vi "Read_Traverse_Space_Size.vi"(1 "Space_Name":string, 2 "Traverse Name":string) -> (0 "Limits out":T1=[{"Max"=15.0, "Min"=-15.0}, {"Max"=250.0, "Min"=0.0}, {"Max"=15.0, "Min"=-15.0}] {"Min" format="%#.1f"; "Max" format="%#.1f"})   [LabVIEW 2022 SP3]
uses:
  Route mapping/Box_size.ctl
  Globals/Constants_global.vi
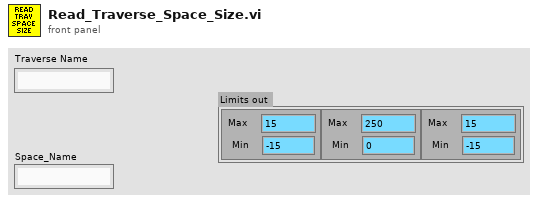
[diagram p1: front panel]
types:
  T1 = typedef "Box_size.ctl" = cluster{"Max":sgl, "Min":sgl}[]
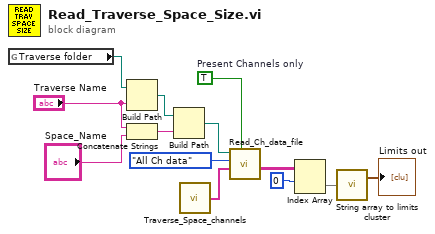
[diagram p0: block diagram]
diagram:
  w8 = TRUE  # Present Channels only
  n1 = global read "Constants_global.vi" "Traverse folder"() -> (w6:path)
  n2 = Build Path(base path=w6, name or relative path="Traverse Name") -> (appended path=w5:path)
  n3 = Concatenate Strings("Traverse Name", "Space_Name") -> (w9:string)
  n4 = Build Path(base path=w5, name or relative path=w9) -> (appended path=w10:path)
  n5 = call "Traverse_Space_channels.vi"() -> ("Channel Names"=w3:string[])
  n6 = call "Read_Ch_data_file.vi"("Present Channels only"=w8, "Present Channels"=w3, "Output"=enum16{"All Ch data", "The last few rows"}."All Ch data", "Filename"=w10) -> ("Channel Values"=w11:string[][])  [unwired: 1 in, 4 out]
  n7 = Index Array(array=w11, index (row)=0) -> (element=w13:string[])  [unwired: 1 in]
  n8 = call "String array to limits cluster.vi"("Channel Values in"=w13) -> ("Limits out"=→"Limits out":T1)  [unwired: 1 out]
